vi "ISE_interface.vi"() -> ()   [LabVIEW 2011]
uses:
  <vilib>/DAQmx/read.llb/DAQmx Read (Analog DBL 1Chan 1Samp).vi
  <vilib>/DAQmx/create/channels.llb/DAQmx Create Channel (AI-Voltage-Basic).vi
  <vilib>/DAQmx/miscellaneous.llb/DAQmx Fill In Error Info.vi
  <vilib>/ptbypt/NI_PtbyPt.lvlib
panel:
  in  "sample length":i32=100
  out "mean":dbl(graph)
  in  "stop":bool
  out "data":dbl(graph)
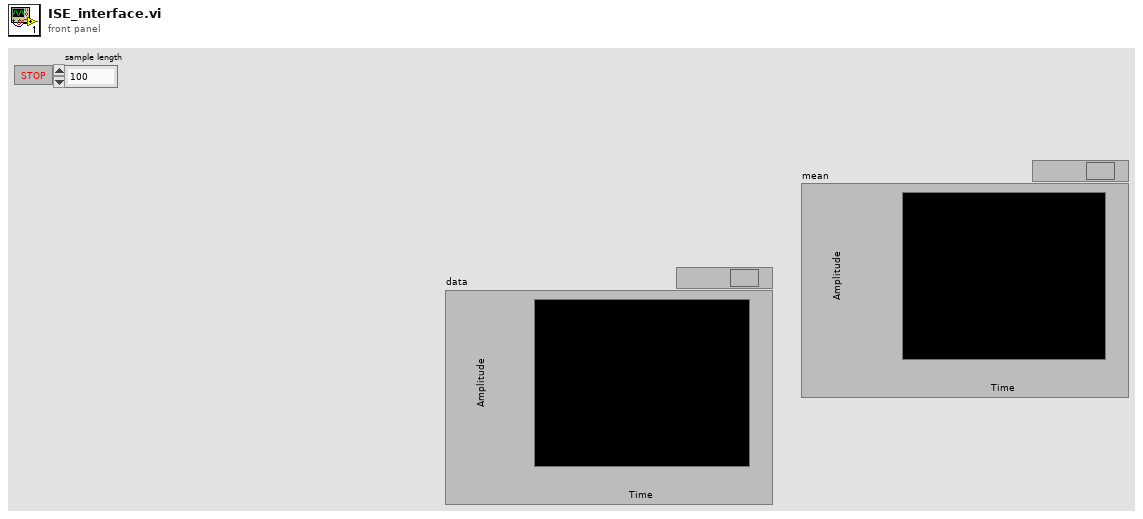
[diagram p1: front panel]
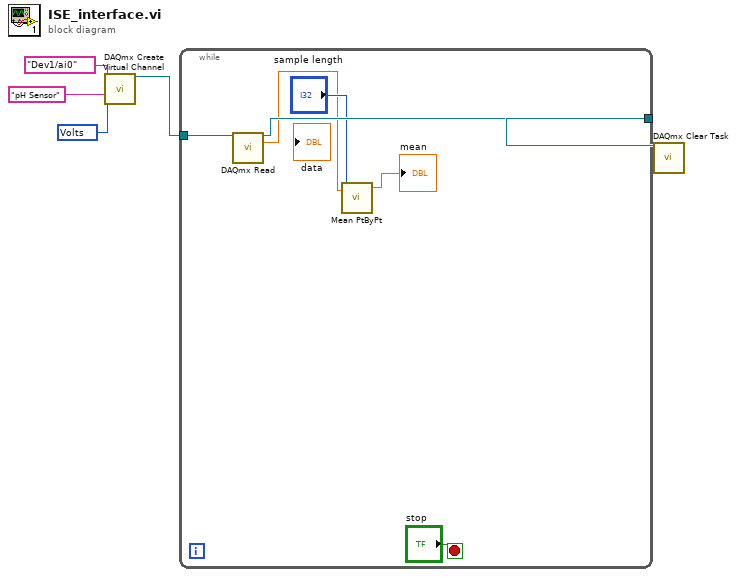
[diagram p0: block diagram]
diagram:
  w3 = 10348 items=["Volts"=10348, "From Custom Scale"=10065] ("units")
  n1 = call-poly <vilib>:"DAQmx Create Virtual Channel.vi"("physical channels"=tag "Dev1/ai0", "name to assign"="pH Sensor", "units"=w3) -> ("task out"=w2:refnum<k21>)  [unwired: 11 in, 1 out]
  n2 = while {
    tunnel: w2 -> [w11]
    tunnel: [w9] -> w1
    stop <- "stop" stop-if-true
    n3 = call-poly <vilib>:"DAQmx Read.vi"("task/channels in"=w11) -> ("task out"=w9:refnum<k21>, "data"=w6:dbl)  [unwired: 12 in, 1 out]
    n4 = call <vilib>:"Mean PtByPt.vi"("x"=w6, "sample length"="sample length") -> ("mean"=→"mean":dbl)  [unwired: 2 in, 1 out]
  }
  n5 = call <vilib>:"DAQmx Clear Task.vi"("task in"=w1) -> ()  [unwired: 14 in, 1 out]
